vi "Example_Calib_MHM.vi"() -> ()   [LabVIEW 2019]
panel:
  in  "error in (no error)":errorcluster
  in  "pulMHMHandle":u32
  out "Revolutions":dbl step=1.0
  out "Error_bit":dbl caption="bit" format="%.03f%.;"
  out "Error Range":dbl caption="degree" format="%.03f%.;"
  out "XY Graph":cluster{dbl[], dbl[]}[](graph) caption="Calibration Curves"
  in  "Number of Samples":u32=1000 min=1 max=15000 step=1
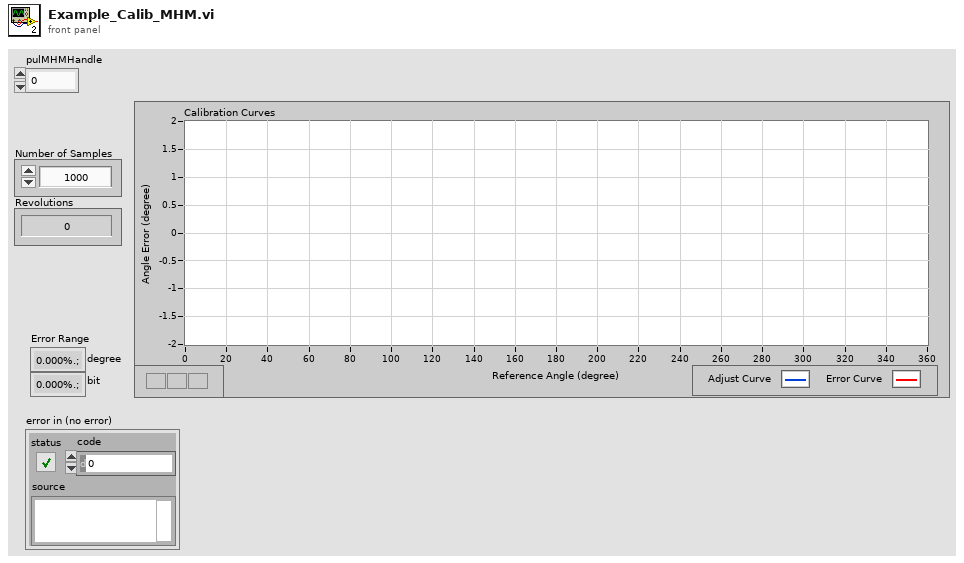
[diagram p1: front panel]
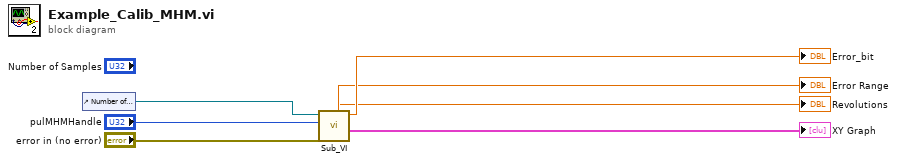
[diagram p0: block diagram]
diagram:
  n1 = control-ref of="Number of Samples"() -> (w7:refnum<vi>)
  n2 = call "Sub_VI.vi"("error in (no error)"="error in (no error)", "pulMHMHandle"="pulMHMHandle", "Digital in"=w7) -> ("XY Graph"=→"XY Graph":cluster{dbl[], dbl[]}[], "Error Range"=→"Error Range":dbl, "Error_bit"=→"Error_bit":dbl, "Revolutions"=→"Revolutions":dbl)  [unwired: 4 in, 1 out]
